vi "Servo Tracking State Machine.vi"(0 "Servo Positions In":cluster{"X":dbl, "Y":dbl}, 1 "Image Size":T4=enum."320x240", 7 "Rectangle":T3, 9 "Particles":i32, 11 "Area":i32=4) -> (4 "Servo Positions":cluster{"X":dbl, "Y":dbl}, 6 "Tracking State Info":T2)   [LabVIEW 2011]
uses:
  <vilib>/Rock Robotics/WPI/Camera/WPI_CameraImageSize.ctl
  Control States.ctl
panel:
  in  "Upper Limit":cluster{"X":i32, "Y":i32}={"X"=169, "Y"=130}
  in  "Lower Limit":cluster{"X":i32, "Y":i32}={"X"=0, "Y"=40}
  in  "Search Speed":i32=4
  in  "Proportional (div)":cluster{"X":i32, "Y":i32}={"X"=15, "Y"=-13}
  # "Unwired tuning params for control.\nSearch speed determines how fast the\ngimbal will move when trying to acquire\na target. Too fast and you may miss the\ntarget between frames, too slow is boring.\n\nProportional(div) is the proportional constant\nexpressed as a divisor term. Adjust this higher\nif the gimbal is oscillating, lower for quicker\nresponse.\n\nThe limits are useful for keeping the gimbal in\na working range, some stick when the get near\ntheir mechanical limits. It is also useful to limit\nthe searching to avoid looking at the ceiling, etc."
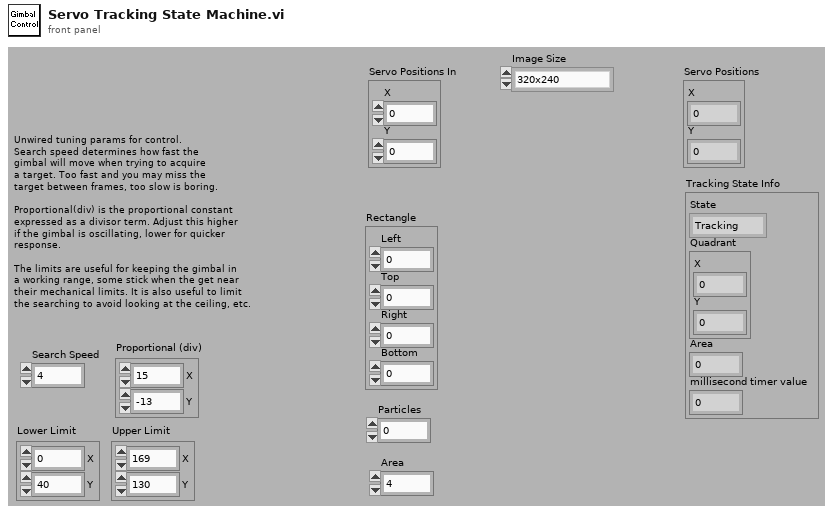
[diagram p1: front panel]
types:
  T1 = typedef "Control States.ctl" = enum16{"Tracking", "Lost Small", "Lost-Patience", "Search-Begin", "Searching", "Lost - Edge"}
  T2 = cluster{"State":T1, "Quadrant":cluster{"X":i32, "Y":i32}, "Area":i32, "millisecond timer value":u32}
  T3 = cluster{"Left":i32, "Top":i32, "Right":i32, "Bottom":i32}
  T4 = typedef "WPI_CameraImageSize.ctl" = enum16{"640x480", "320x240", "160x120"}
  T5 = cluster{"State":T1, "Grid Element":cluster{"X":i32, "Y":i32}, "Area":i32, "millisecond timer value":u32}
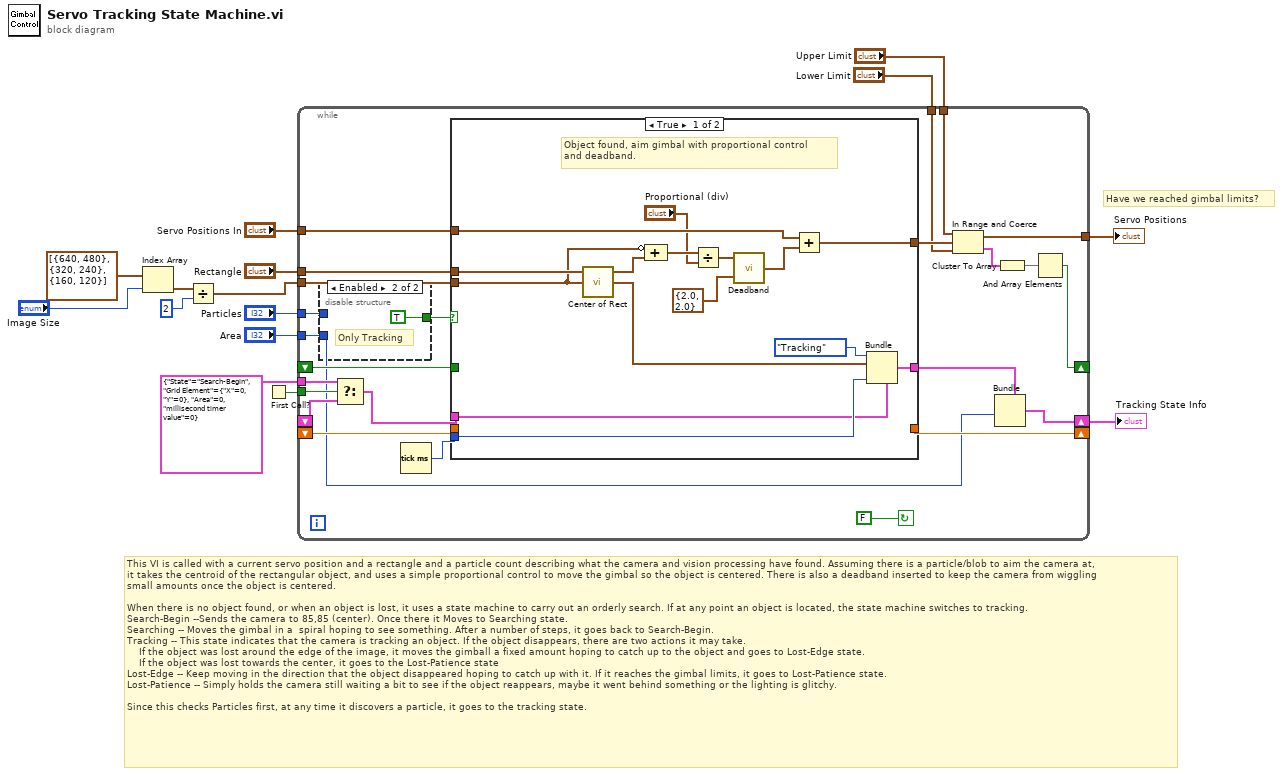
[diagram p0: block diagram]
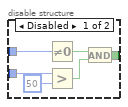
[diagram p2: hidden frame]
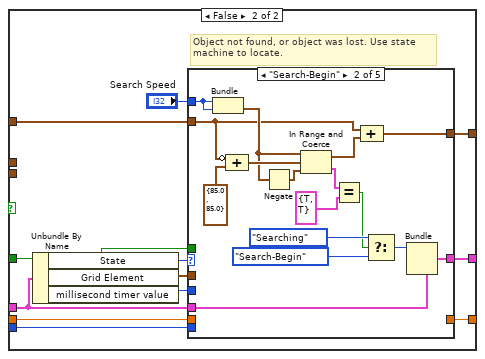
[diagram p3: hidden frame]
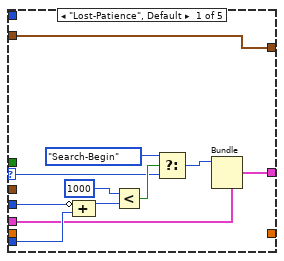
[diagram p4: hidden frame]
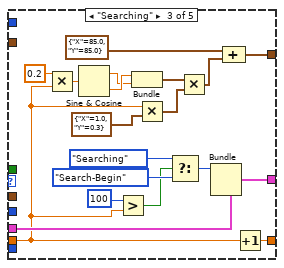
[diagram p5: hidden frame]
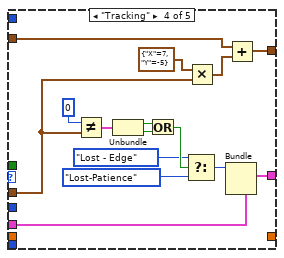
[diagram p6: hidden frame]
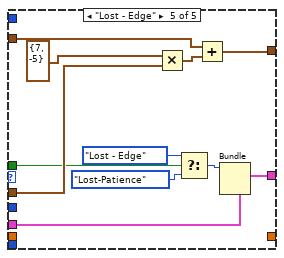
[diagram p7: hidden frame]
diagram:
  # "Have we reached gimbal limits?"
  # "This VI is called with a current servo position and a rectangle and a particle count describing what the camera and vision processing have found. Assuming there is a particle/blob to aim the camera at,\nit takes the centroid of the rectangular object, and uses a simple proportional control to move the gimbal so the object is centered. There is also a deadband inserted to keep the camera from wiggling\nsmall amounts once the object is centered.\n\nWhen there is no object found, or when an object is lost, it uses a state machine to carry out an orderly search. If at any point an object is located, the state machine switches to tracking.\nSearch-Begin --Sends the camera to 85,85 (center). Once there it Moves to Searching state.\nSearching -- Moves the gimbal in a  spiral hoping to see something. After a number of steps, it goes back to Search-Begin.\nTracking -- This state indicates that the camera is tracking an object. If the object disappears, there are two actions it may take.\n    If the object was lost around the edge of the image, it moves the gimball a fixed amount hoping to catch up to the object and goes to Lost-Edge state.\n    If the object was lost towards the center, it goes to the Lost-Patience state\nLost-Edge -- Keep moving in the direction that the object disappeared hoping to catch up with it. If it reaches the gimbal limits, it goes to Lost-Patience state.\nLost-Patience -- Simply holds the camera still waiting a bit to see if the object reappears, maybe it went behind something or the lighting is glitchy.\n\nSince this checks Particles first, at any time it discovers a particle, it goes to the tracking state."
  n1 = Index Array(array=cluster{"X":i32, "Y":i32}[] [{"X"=640, "Y"=480}, {"X"=320, "Y"=240}, {"X"=160, "Y"=120}] ("Resolutions"), index="Image Size") -> (element=w12:cluster{"X":i32, "Y":i32})
  n2 = Divide(x=w12, y=2) -> (x/y=w13:cluster{"X":dbl, "Y":dbl})
  n3 = First Call?() -> (First Call?: T/F=w5:bool)
  n4 = while {
    tunnel: w13 -> [w21]
    tunnel: "Particles" -> [w20]
    tunnel: "Rectangle" -> [w22]
    tunnel: [w30] -> w8
    shift-right: [w38] -> _
    shift-left: _ -> [w37]
    tunnel: "Servo Positions In" -> [w36]
    shift-right: [w18] -> w6
    shift-left: _ -> [w33]
    tunnel: w5 -> [w35]
    tunnel: T5 {"State"=enum."Search-Begin", "Grid Element"={"X"=0, "Y"=0}, "Area"=0, "millisecond timer value"=0} -> [w34]
    tunnel: "Lower Limit" -> [w28]
    tunnel: "Upper Limit" -> [w27]
    shift-right: [w24] -> _
    shift-left: _ -> [w23]
    tunnel: "Area" -> [w16]
    stop <- FALSE continue-if-true
    n5 = disable-structure shown="Enabled" {
      disable-tunnel: w20 -> [w45 _]
      disable-tunnel: [w41 TRUE] -> w19
      disable-tunnel: w16 -> [w40 _]
      frame Disabled {
        n6 = Not Equal To 0?(x=w45) -> (x != 0?=w43:bool)
        n7 = Greater?(x=w40, y=50) -> (0:w42:bool)
        n8 = And(x=w43, y=w42) -> (x .and. y?=w41:bool)
      }
      frame Enabled {
        # "Only Tracking"
      }
    }
    n9 = Select(t=w34, s=w35, f=w33) -> (s? t:f=w32:T5)
    n10 = Tick Count (ms)() -> (millisecond timer value=w39:u32)
    n11 = case shown="True" w19 {
      tunnel: w22 -> [w50 _]
      tunnel: w21 -> [w47 _]
      tunnel: w39 -> [w57 w72]
      tunnel: [w59 w73] -> w17
      tunnel: w32 -> [w51 w65]
      tunnel: w36 -> [w58 w70]
      tunnel: [w56 w71] -> w29
      tunnel: w37 -> [_ w69]
      tunnel: [_ w68] -> w38
      tunnel: w23 -> [_ w67]
      frame True {
        # "Object found, aim gimbal with proportional control\nand deadband."
        n12 = call "Center of Rect.vi"("Camera Center"=w47, "Rectangle"=w50) -> ("Grid Element"=w48:cluster{"X":i32, "Y":i32}, "Center"=w49:cluster{dbl, dbl})  [unwired: 1 in, 1 out]
        n13 = Compound Arithmetic op=ADD(invert w47, w49) -> (w61:cluster{dbl, dbl})
        n14 = Divide(x=w61, y="Proportional (div)") -> (x/y=w54:cluster{dbl, dbl})
        n15 = call "Deadband.vi"("Deadband"=cluster{dbl, dbl} {2.0, 2.0}, "Value"=w54) -> ("Value Out"=w53:cluster{dbl, dbl})
        n16 = Add(x=w58, y=w53) -> (x+y=w56:cluster{dbl, dbl})
        n17 = Bundle(cluster=w51, "State"=Control_States."Tracking", "Grid Element"=w48, "millisecond timer value"=w57) -> (w59:T5)  [unwired: 1 out]
      }
      frame False {
        # "Object not found, or object was lost. Use state\nmachine to locate."
        n18 = Unbundle By Name(w65) -> ("State"=w64:T1, "Grid Element"=w63:cluster{"X":i32, "Y":i32}, "millisecond timer value"=w62:u32)
        n19 = case shown="\"Search-Begin\"" w64 {
          selector: w64 -> [w75 _ _ _ _]
          tunnel: [w76 w91 w106 w134 w145] -> w73
          tunnel: w65 -> [w80 w92 w107 w133 w144]
          tunnel: w62 -> [w83 _ _ _ _]
          tunnel: w72 -> [w84 _ _ _ _]
          tunnel: [w74 w93 w111 w125 w140] -> w71
          tunnel: w70 -> [w74 w94 _ w124 w141]
          tunnel: "Search Speed" -> [_ w98 _ _ _]
          tunnel: w69 -> [_ _ w102 _ _]
          tunnel: [_ _ w119 _ _] -> w68
          tunnel: w63 -> [_ _ _ w121 w139]
          tunnel: w67 -> [_ _ _ _ w135]
          frame "Lost-Patience", Default {
            n20 = Compound Arithmetic op=ADD(invert w83, w84) -> (w82:u32)
            n21 = Less?(x=1000, y=w82) -> (x < y?=w77:bool)
            n22 = Select(t=Control_States."Search-Begin" ("State"), s=w77, f=w75) -> (s? t:f=w79:T1)
            n23 = Bundle(cluster=w80, "State"=w79) -> (w76:T5)  [unwired: 3 out]
          }
          frame "Search-Begin" {
            n24 = Bundle("Search Speed"=w98, "Search Speed"=w98) -> (w97:cluster{"Search Speed":i32, "Search Speed":i32})  [unwired: 1 out]
            n25 = Compound Arithmetic op=ADD(invert w94, cluster{"X":dbl, "Y":dbl} {"X"=85.0, "Y"=85.0} ("Servos")) -> (w99:cluster{"X":dbl, "Y":dbl})
            n26 = Negate(x=w97) -> (-x=w96:cluster{"Search Speed":i32, "Search Speed":i32})
            n27 = In Range and Coerce(upper limit=w97, x=w99, lower limit=w96) -> (coerced(x)=w95:cluster{"X":dbl, "Y":dbl}, In Range?=w87:cluster{"X":bool, "Y":bool})
            n28 = Equal?(x=w87, y=cluster{"X":bool, "Y":bool} {"X"=TRUE, "Y"=TRUE}) -> (x = y?=w85:bool)
            n29 = Compound Arithmetic op=ADD(w94, w95) -> (w93:cluster{"X":dbl, "Y":dbl})
            n30 = Select(t=Control_States."Searching" ("State"), s=w85, f=Control_States."Search-Begin" ("State")) -> (s? t:f=w90:T1)
            n31 = Bundle(cluster=w92, "State"=w90) -> (w91:T5)  [unwired: 3 out]
          }
          frame "Searching" {
            n32 = Multiply(x=0.2, y=w102) -> (x*y=w117:dbl)
            n33 = Sine & Cosine(0:w117) -> (1:w115:dbl, 2:w116:dbl)
            n34 = Greater?(x=100, y=w102) -> (0:w104:bool)
            n35 = Bundle(w116, w115) -> (w114:cluster{dbl, dbl})  [unwired: 1 out]
            n36 = Multiply(x=w102, y=cluster{"X":dbl, "Y":dbl} {"X"=1.0, "Y"=0.3} ("Servos")) -> (x*y=w103:cluster{"X":dbl, "Y":dbl})
            n37 = Select(t=Control_States."Searching" ("State"), s=w104, f=Control_States."Search-Begin" ("State")) -> (s? t:f=w110:T1)
            n38 = Multiply(x=w114, y=w103) -> (x*y=w113:cluster{dbl, dbl})
            n39 = Bundle(cluster=w107, "State"=w110) -> (w106:T5)  [unwired: 3 out]
            n40 = Compound Arithmetic op=ADD(cluster{"X":dbl, "Y":dbl} {"X"=85.0, "Y"=85.0} ("Servos"), w113) -> (w111:cluster{dbl, dbl})
            n41 = Increment(x=w102) -> (x+1=w119:dbl)
          }
          frame "Tracking" {
            n42 = Not Equal?(x=0 ("X"), y=w121) -> (x != y?=w132:cluster{"X":bool, "Y":bool})
            n43 = Unbundle(w132) -> ("X"=w131:bool, "Y"=w130:bool)
            n44 = Or(x=w131, y=w130) -> (x .or. y?=w129:bool)
            n45 = Select(t=Control_States."Lost - Edge" ("State"), s=w129, f=Control_States."Lost-Patience" ("State")) -> (s? t:f=w126:T1)
            n46 = Multiply(x=cluster{"X":i32, "Y":i32} {"X"=7, "Y"=-5}, y=w121) -> (x*y=w123:cluster{"X":i32, "Y":i32})
            n47 = Bundle(cluster=w133, "State"=w126) -> (w134:T5)  [unwired: 3 out]
            n48 = Add(x=w124, y=w123) -> (x+y=w125:cluster{"X":dbl, "Y":dbl})
          }
          frame "Lost - Edge" {
            n49 = Multiply(x=cluster{"X":i32, "Y":i32} {"X"=7, "Y"=-5}, y=w139) -> (x*y=w143:cluster{"X":i32, "Y":i32})
            n50 = Select(t=Control_States."Lost - Edge" ("State"), s=w135, f=Control_States."Lost-Patience" ("State")) -> (s? t:f=w138:T1)
            n51 = Add(x=w141, y=w143) -> (x+y=w140:cluster{"X":dbl, "Y":dbl})
            n52 = Bundle(cluster=w144, "State"=w138) -> (w145:T5)  [unwired: 3 out]
          }
        }
      }
    }
    n53 = In Range and Coerce(upper limit=w27, x=w29, lower limit=w28) -> (coerced(x)=w30:cluster{"X":dbl, "Y":dbl}, In Range?=w26:cluster{"X":bool, "Y":bool})
    n54 = Bundle(cluster=w17, "Area"=w16) -> (w18:T5)  [unwired: 3 out]
    n55 = Cluster To Array(cluster=w26) -> (array=w25:bool[])
    n56 = And Array Elements(Boolean array=w25) -> (logical AND=w24:bool)
  }
  "Servo Positions" <- w8
  "Tracking State Info" <- w6
